vi "Sample Encoder DMA.vi"(8 "error in (no error)":T1) -> (0 "error out":T1, 3 "Array":T2)   [LabVIEW 2019]
uses:
  <vilib>/Utility/error.llb/Error Cluster From Error Code.vi
  <vilib>/rvi/errors/niLvFpgaAdjustHostInterfaceError.vi
  <vilib>/rvi/interface/nirviMethod/nirviMethod.xnode
  <vilib>/Rock Robotics/SystemInterfaces/System/FPGA_SystemFRC FPGA Ref.ctl
  <vilib>/FPGAPlugInAG/Dynamic/niLvFpga_ReadFifo_Dynamic.vi
  <vilib>/rvi/errors/niLvFpgaMergeErrorWithErrorCode.vi
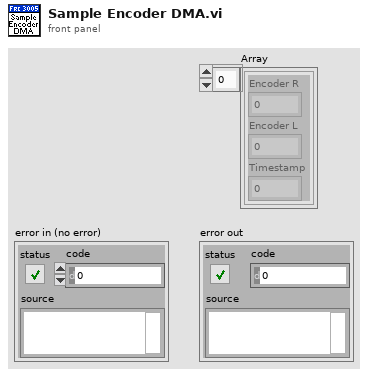
[diagram p1: front panel]
types:
  T1 = cluster{"source":string, "code":numeric, "status":boolean}
  T2 = array[cluster{"Encoder R":numeric, "Encoder L":numeric, "Timestamp":numeric}]
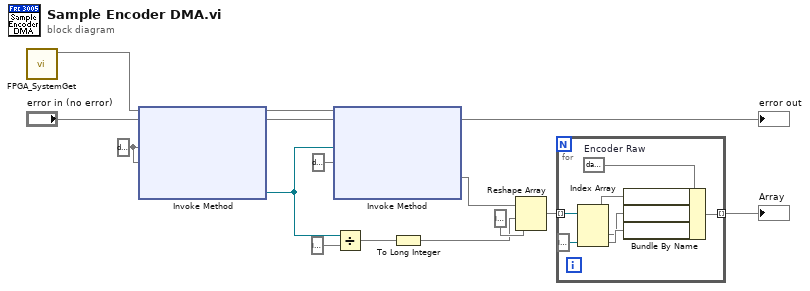
[diagram p0: block diagram]
diagram:
  w7 = data[5B] ("Number of Elements")
  n1 = call <vilib>:"FPGA_SystemGet.vi"() -> (3:w1)  [unwired: 11 in]
  n2 = xnode "Invoke Method"(w1, "error in (no error)", w7, w7) -> (w6, w5, w3)  [unwired: 1 out]
  n3 = xnode "Invoke Method"(w6, w5, w3, data[5B] ("Timeout (ms)")) -> (→"error out", w10)  [unwired: 2 out]
  n4 = Divide(x=w3, y=i32? 5) -> (x/y=w12)
  n5 = To Long Integer(number=w12) -> (32bit integer=w13)
  n6 = Reshape Array(w10, w13, i32? 5 ("dimension size")) -> (w15)
  n7 = for {
    tunnel: w15 -> [w21] mode=indexing
    tunnel: [w16] -> w8 mode=indexing
    w22 = data[13B]  # Encoder Raw
    n8 = Index Array(array=w21, index #3=i32? 4 ("index")) -> (element #1=w17, element #2=w18, element #3=w19)  [unwired: 2 in]
    n9 = Bundle By Name(cluster=w22, w17, w18, w19) -> (w16)
  }
  "Array" <- w8
